vi "Connecting_Indicator(SubVI).vi"(10 "Numeric":dbl, 11 "Numeric 2":dbl) -> (1 "f":dbl, 2 "f 2":dbl, 3 "String":string="Подключение.", 5 "Slide":u8(slide) scale=0.0..100.0)   [LabVIEW 2017]
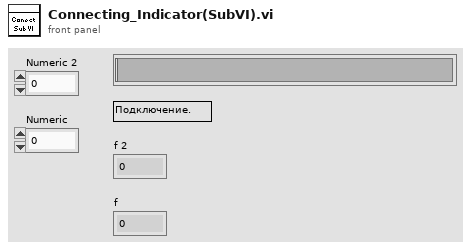
[diagram p1: front panel]
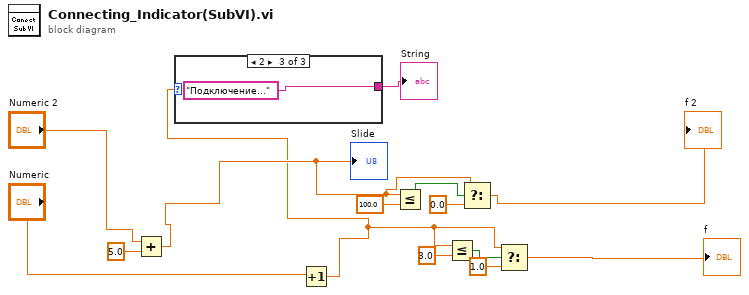
[diagram p0: block diagram]
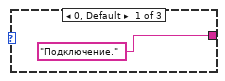
[diagram p2: hidden frame]
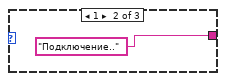
[diagram p3: hidden frame]
diagram:
  n1 = Add(x="Numeric 2", y=5.0) -> (x+y=w14:dbl)
  "Slide" <- w14
  n2 = Increment(x="Numeric") -> (x+1=w9:dbl)
  n3 = case shown="2" w9 {
    tunnel: ["Подключение." ("String") "Подключение.." ("String") "Подключение..." ("String")] -> w7
    frame 0, Default {
    }
    frame 1 {
    }
    frame 2 {
    }
  }
  "String" <- w7
  n4 = Less Or Equal?(x=w14, y=100.0) -> (x <= y?=w4:bool)
  n5 = Less Or Equal?(x=w9, y=3.0) -> (x <= y?=w11:bool)
  n6 = Select(t=w14, s=w4, f=0.0) -> (s? t:f=→"f 2":dbl)
  n7 = Select(t=w9, s=w11, f=1.0) -> (s? t:f=→"f":dbl)
